vi "GetSupportedFunctions.vi"(11 "package":path=path "C:/Users/Darin/Documents/pyVI/src/pyVI") -> (1 "Functions":T1, 3 "Functions":variant)   [LabVIEW 2014, in "Raspberry Pi Compatible Compiler for LabVIEW.lvlib" / "Python Functions.lvlib"]
uses:
  Python Functions.lvlib
  FunctionsTD.ctl
  DocstringTD.ctl
  Classes/PythonFunction/PythonFunction.lvclass/PythonFunction.ctl
  Classes/PythonFunction/PythonFunction.lvclass
  <vilib>/Utility/file.llb/Write To Spreadsheet File (string).vi
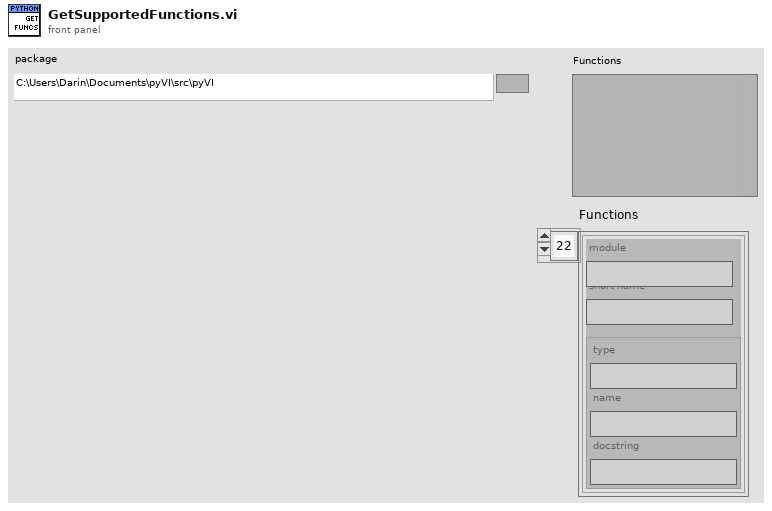
[diagram p1: front panel]
types:
  T1 = typedef "Raspberry Pi Compatible Compiler for LabVIEW.lvlib/Python Functions.lvlib/FunctionsTD.ctl" = cluster{"module":string, "short name":string, "docstrings":T2}[]
  T2 = typedef "Raspberry Pi Compatible Compiler for LabVIEW.lvlib/Python Functions.lvlib/DocstringTD.ctl" = cluster{"type":string, "name":string, "docstring":string}
  T3 = cluster{"module":string, "short name":string, "docstrings":T2}
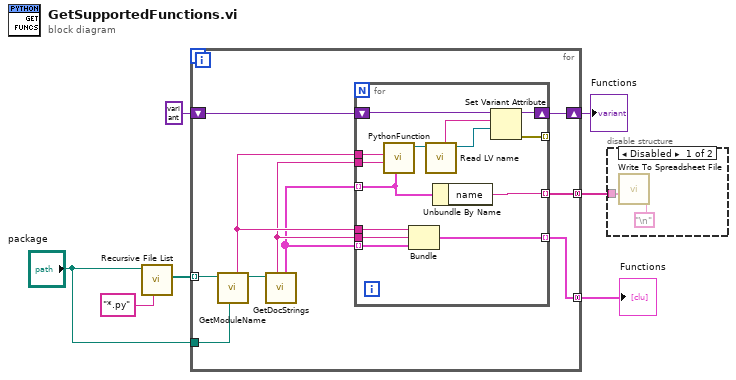
[diagram p0: block diagram]
diagram:
  n1 = call <vilib>:"Recursive File List.vi"("pattern"="*.py", "Folder Path"="package") -> ("All Files in Dir"=w6:path[])  [unwired: 5 in, 4 out]
  n2 = for {
    tunnel: w6 -> [w17] mode=indexing
    tunnel: "package" -> [w16]
    shift-right: [w13] -> w3
    shift-left: variant -> [w14]
    tunnel: [w12] -> w2 mode=concatenating
    tunnel: [w8] -> w1 mode=concatenating
    n3 = call "GetModuleName.vi"("package"=w16, "path in"=w17) -> ("path out"=w15:path, "module"=w11:string)  [unwired: 6 in]
    n4 = call "GetDocStrings.vi"("path in"=w15) -> ("docstrings"=w9:T2[], "short name"=w10:string)  [unwired: 5 in, 2 out]
    n5 = for {
      tunnel: w11 -> [w31]
      tunnel: w10 -> [w30]
      tunnel: w9 -> [w24] mode=indexing
      shift-right: [w28] -> w13
      shift-left: w14 -> [w27]
      tunnel: [w23] -> w12 mode=indexing
      tunnel: w11 -> [w22]
      tunnel: w10 -> [w21]
      tunnel: w9 -> [w20] mode=indexing
      tunnel: [w19] -> w8 mode=indexing
      tunnel: [w18] -> _ mode=indexing
      n6 = call "PythonFunction.vi"("info"=w24, "Python module  name"=w30, "Python module"=w31) -> ("PythonFunction out"=w29:refnum<class "PythonFunction.lvclass">)  [unwired: 8 in]
      n7 = Bundle("module"=w22, "short name"=w21, "docstrings"=w20) -> (w19:T3)  [unwired: 1 in]
      n8 = call "Read LV name.vi"("PythonFunction in"=w29) -> ("PythonFunction out"=w25:refnum<class "PythonFunction.lvclass">, "LV name"=w26:string)  [unwired: 7 in]
      n9 = Unbundle By Name(w24) -> ("name"=w23:string)
      n10 = Set Variant Attribute(Variant=w27, name=w26, value=w25) -> (Variant out=w28:variant, error out=w18:errorcluster)  [unwired: 1 in, 1 out]
    }
  }
  "Functions" <- w3
  "Functions" <- w1
  n11 = disable-structure shown="Disabled" {
    disable-tunnel: w2 -> [w33 _]
    frame Disabled {
      n12 = call-poly <vilib>:"Write To Spreadsheet File.vi"("delimiter (\\t)"="\n", "1D data"=w33) -> ()  [unwired: 6 in, 1 out]
    }
    frame Enabled {
    }
  }
